vi "create.vi"(5 "history":u64, 7 "uid":u64, 8 "error in (no error)":errorcluster, 11 "PersistentObject in":refnum<class "PersistentObject.lvclass">) -> (0 "error out":errorcluster, 3 "PersistentObject out":refnum<class "PersistentObject.lvclass">)   [LabVIEW 2018, in "PersistentObject.lvclass"]
uses:
  PersistentObject.lvclass
  PersistentObject.lvclass/PersistentObject.ctl
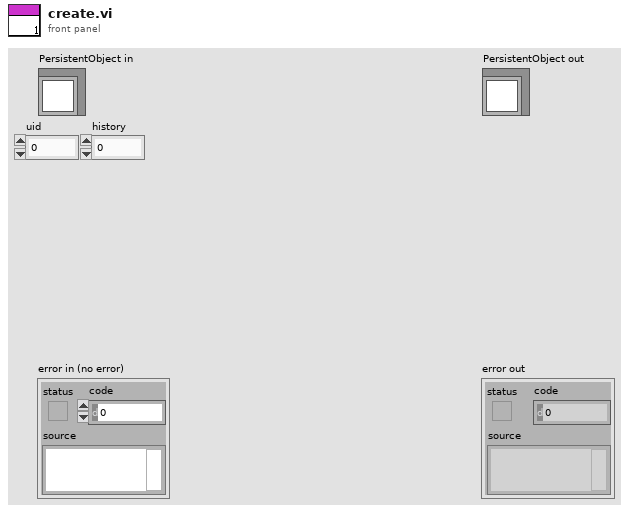
[diagram p1: front panel]
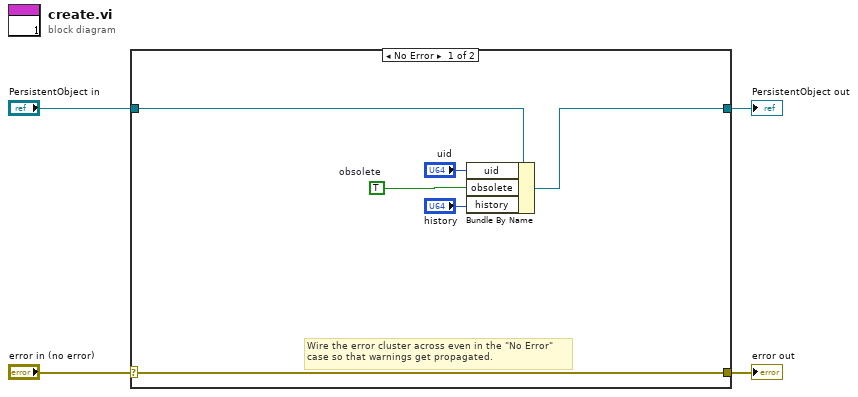
[diagram p0: block diagram]
diagram:
  n1 = case shown="No Error" "error in (no error)" {
    selector: "error in (no error)" -> [w10 w12]
    tunnel: [w10 w12] -> w3
    tunnel: [w9 w11] -> w1
    tunnel: "PersistentObject in" -> [w8 w11]
    frame No Error {
      w5 = TRUE  # obsolete
      # "Wire the error cluster across even in the \"No Error\"\ncase so that warnings get propagated."
      n2 = Bundle By Name(cluster=w8, "uid"="uid", "obsolete"=w5, "history"="history") -> (w9:refnum<class "PersistentObject.lvclass">)
    }
    frame Error {
    }
  }
  "error out" <- w3
  "PersistentObject out" <- w1
